vi "GEA2 HEWH Standard ERDs.vi"(8 "Error In":errorcluster, 10 "ERD Data Input":T1[](array[typedef]) {"ERD Number" format="%.0x"}, 11 "ERD Data  in":T2 {"ERD Therm Data"."EEV Possition" format="%0.0f"; "ERD Therm Data"."T6" format="%.1f"; "ERD Therm Data"."T2" format="%.1f"; "ERD Therm Data"."T3a" format="%.1f"; "ERD Therm Data"."T3b" format="%.1f"; "ERD Therm Data"."T4" format="%.1f"; "ERD Therm Data"."T5" format="%.1f"; "ERD Therm Data"."Current" format="%.1f"}) -> (0 "Error Out":errorcluster, 2 "ERD Data Output":T1[](array[typedef]) {"ERD Number" format="%.0x"}, 3 "ERD Data  out":T2 {"ERD Therm Data"."EEV Possition" format="%0.0f"; "ERD Therm Data"."T6" format="%.1f"; "ERD Therm Data"."T2" format="%.1f"; "ERD Therm Data"."T3a" format="%.1f"; "ERD Therm Data"."T3b" format="%.1f"; "ERD Therm Data"."T4" format="%.1f"; "ERD Therm Data"."T5" format="%.1f"; "ERD Therm Data"."Current" format="%.1f"})   [LabVIEW 2016]
uses:
  type defs/ERD Read Data Out.ctl
  type defs/HEWH ERD Data.ctl
  type defs/HEWH Faults.ctl
  type defs/HEWH Mixing Valve.ctl
  library/GEA2_Toolkit.lvlib
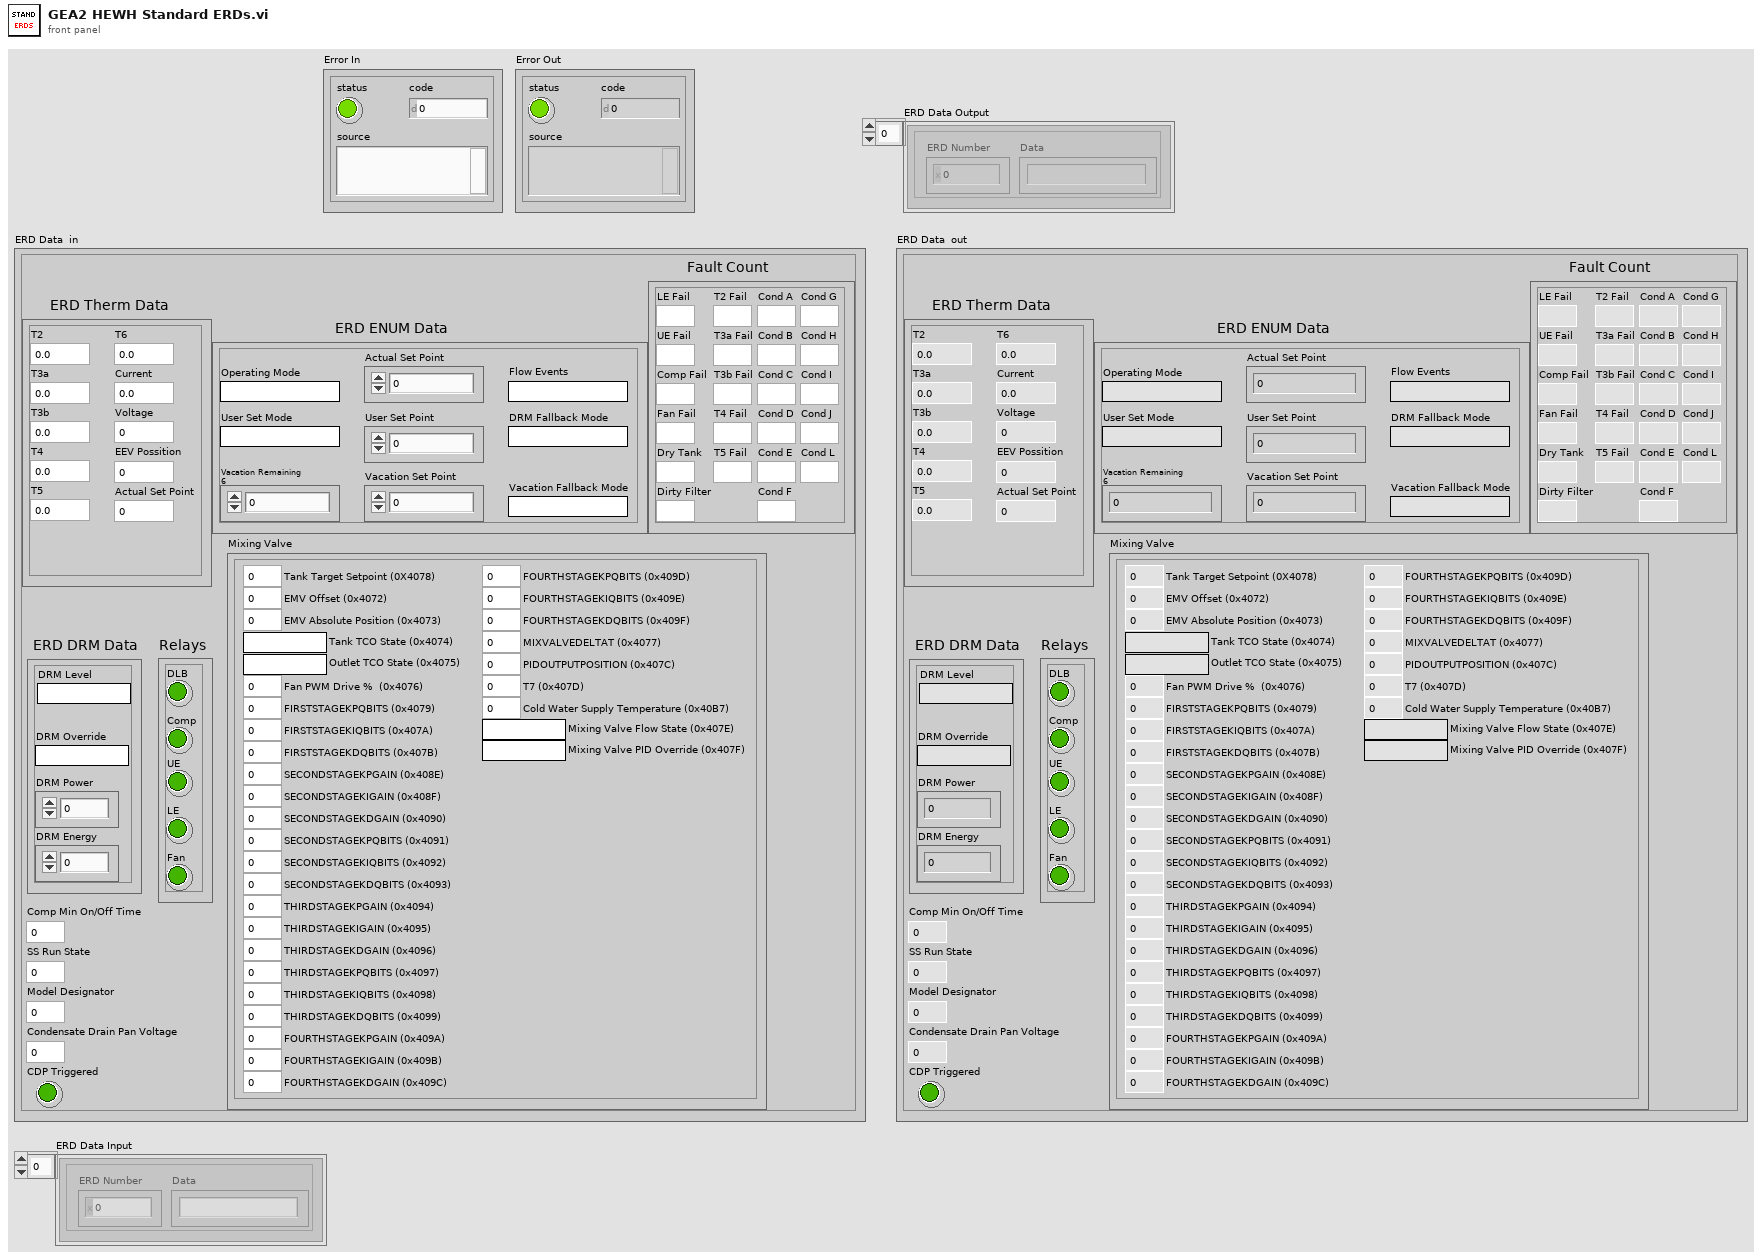
[diagram p1: front panel]
types:
  T1 = typedef "GEA2_Toolkit.lvlib/ERD Read Data Out.ctl" = cluster{"ERD Number":u16, "Data":string}
  T2 = typedef "HEWH ERD Data.ctl" = cluster{"ERD Therm Data":cluster{"T2":dbl, "T3a":dbl, "T3b":dbl, "T4":dbl, "T5":dbl, "T6":dbl, "Current":dbl, "Voltage":dbl, "EEV Possition":dbl, "Actual Set Point":dbl}, "ERD ENUM Data":cluster{"Actual Set Point":dbl, "Flow Events":string, "User Set Mode":string, "Operating Mode":string, "DRM Fallback Mode":string, "Vacation Fallback Mode":string, "User Set Point":dbl, "Vacation Set Point":dbl, "Vacation Remaining\n6":dbl}, "ERD DRM Data":cluster{"DRM Level":string, "DRM Override":string, "DRM Power":dbl, "DRM Energy":dbl}, "Fault Count":T3, "Relays":cluster{"DLB":bool, "Comp":bool, "UE":bool, "LE":bool, "Fan":bool}, "Comp Min On/Off Time":u16, "SS Run State":u16, "Condensate Drain Pan Voltage":u16, "CDP Triggered":bool, "Model Designator":u8, "Mixing Valve":T4}
  T3 = typedef "HEWH Faults.ctl" = cluster{"LE Fail":u32, "UE Fail":u32, "Comp Fail":u32, "T2 Fail":u32, "T3a Fail":u32, "T3b Fail":u32, "T4 Fail":u32, "T5 Fail":u32, "Cond A":u32, "Cond B":u32, "Cond C":u32, "Cond D":u32, "Cond E":u32, "Cond F":u32, "Cond G":u32, "Cond H":u32, "Cond I":u32, "Cond J":u32, "Cond L":u32, "Fan Fail":u32, "Dirty Filter":u32, "Dry Tank":u32}
  T4 = typedef "HEWH Mixing Valve.ctl" = cluster{"Tank Target Setpoint (0X4078)":dbl, "EMV Offset (0x4072)":dbl, "EMV Absolute Position (0x4073)":dbl, "Tank TCO State (0x4074)":string, "Outlet TCO State (0x4075)":string, "Fan PWM Drive %  (0x4076)":dbl, "FIRSTSTAGEKPQBITS (0x4079)":dbl, "FIRSTSTAGEKIQBITS (0x407A)":dbl, "FIRSTSTAGEKDQBITS (0x407B)":dbl, "SECONDSTAGEKPGAIN (0x408E)":dbl, "SECONDSTAGEKIGAIN (0x408F)":dbl, "SECONDSTAGEKDGAIN (0x4090)":dbl, "SECONDSTAGEKPQBITS (0x4091)":dbl, "SECONDSTAGEKIQBITS (0x4092)":dbl, "SECONDSTAGEKDQBITS (0x4093)":dbl, "THIRDSTAGEKPGAIN (0x4094)":dbl, "THIRDSTAGEKIGAIN (0x4095)":dbl, "THIRDSTAGEKDGAIN (0x4096)":dbl, "THIRDSTAGEKPQBITS (0x4097)":dbl, "THIRDSTAGEKIQBITS (0x4098)":dbl, "THIRDSTAGEKDQBITS (0x4099)":dbl, "FOURTHSTAGEKPGAIN (0x409A)":dbl, "FOURTHSTAGEKIGAIN (0x409B)":dbl, "FOURTHSTAGEKDGAIN (0x409C)":dbl, "FOURTHSTAGEKPQBITS (0x409D)":dbl, "FOURTHSTAGEKIQBITS (0x409E)":dbl, "FOURTHSTAGEKDQBITS (0x409F)":dbl, "MIXVALVEDELTAT (0x4077)":dbl, "PIDOUTPUTPOSITION (0x407C)":dbl, "T7 (0x407D)":dbl, "Cold Water Supply Temperature (0x40B7)":dbl, "Mixing Valve Flow State (0x407E)":string, "Mixing Valve PID Override (0x407F)":string}
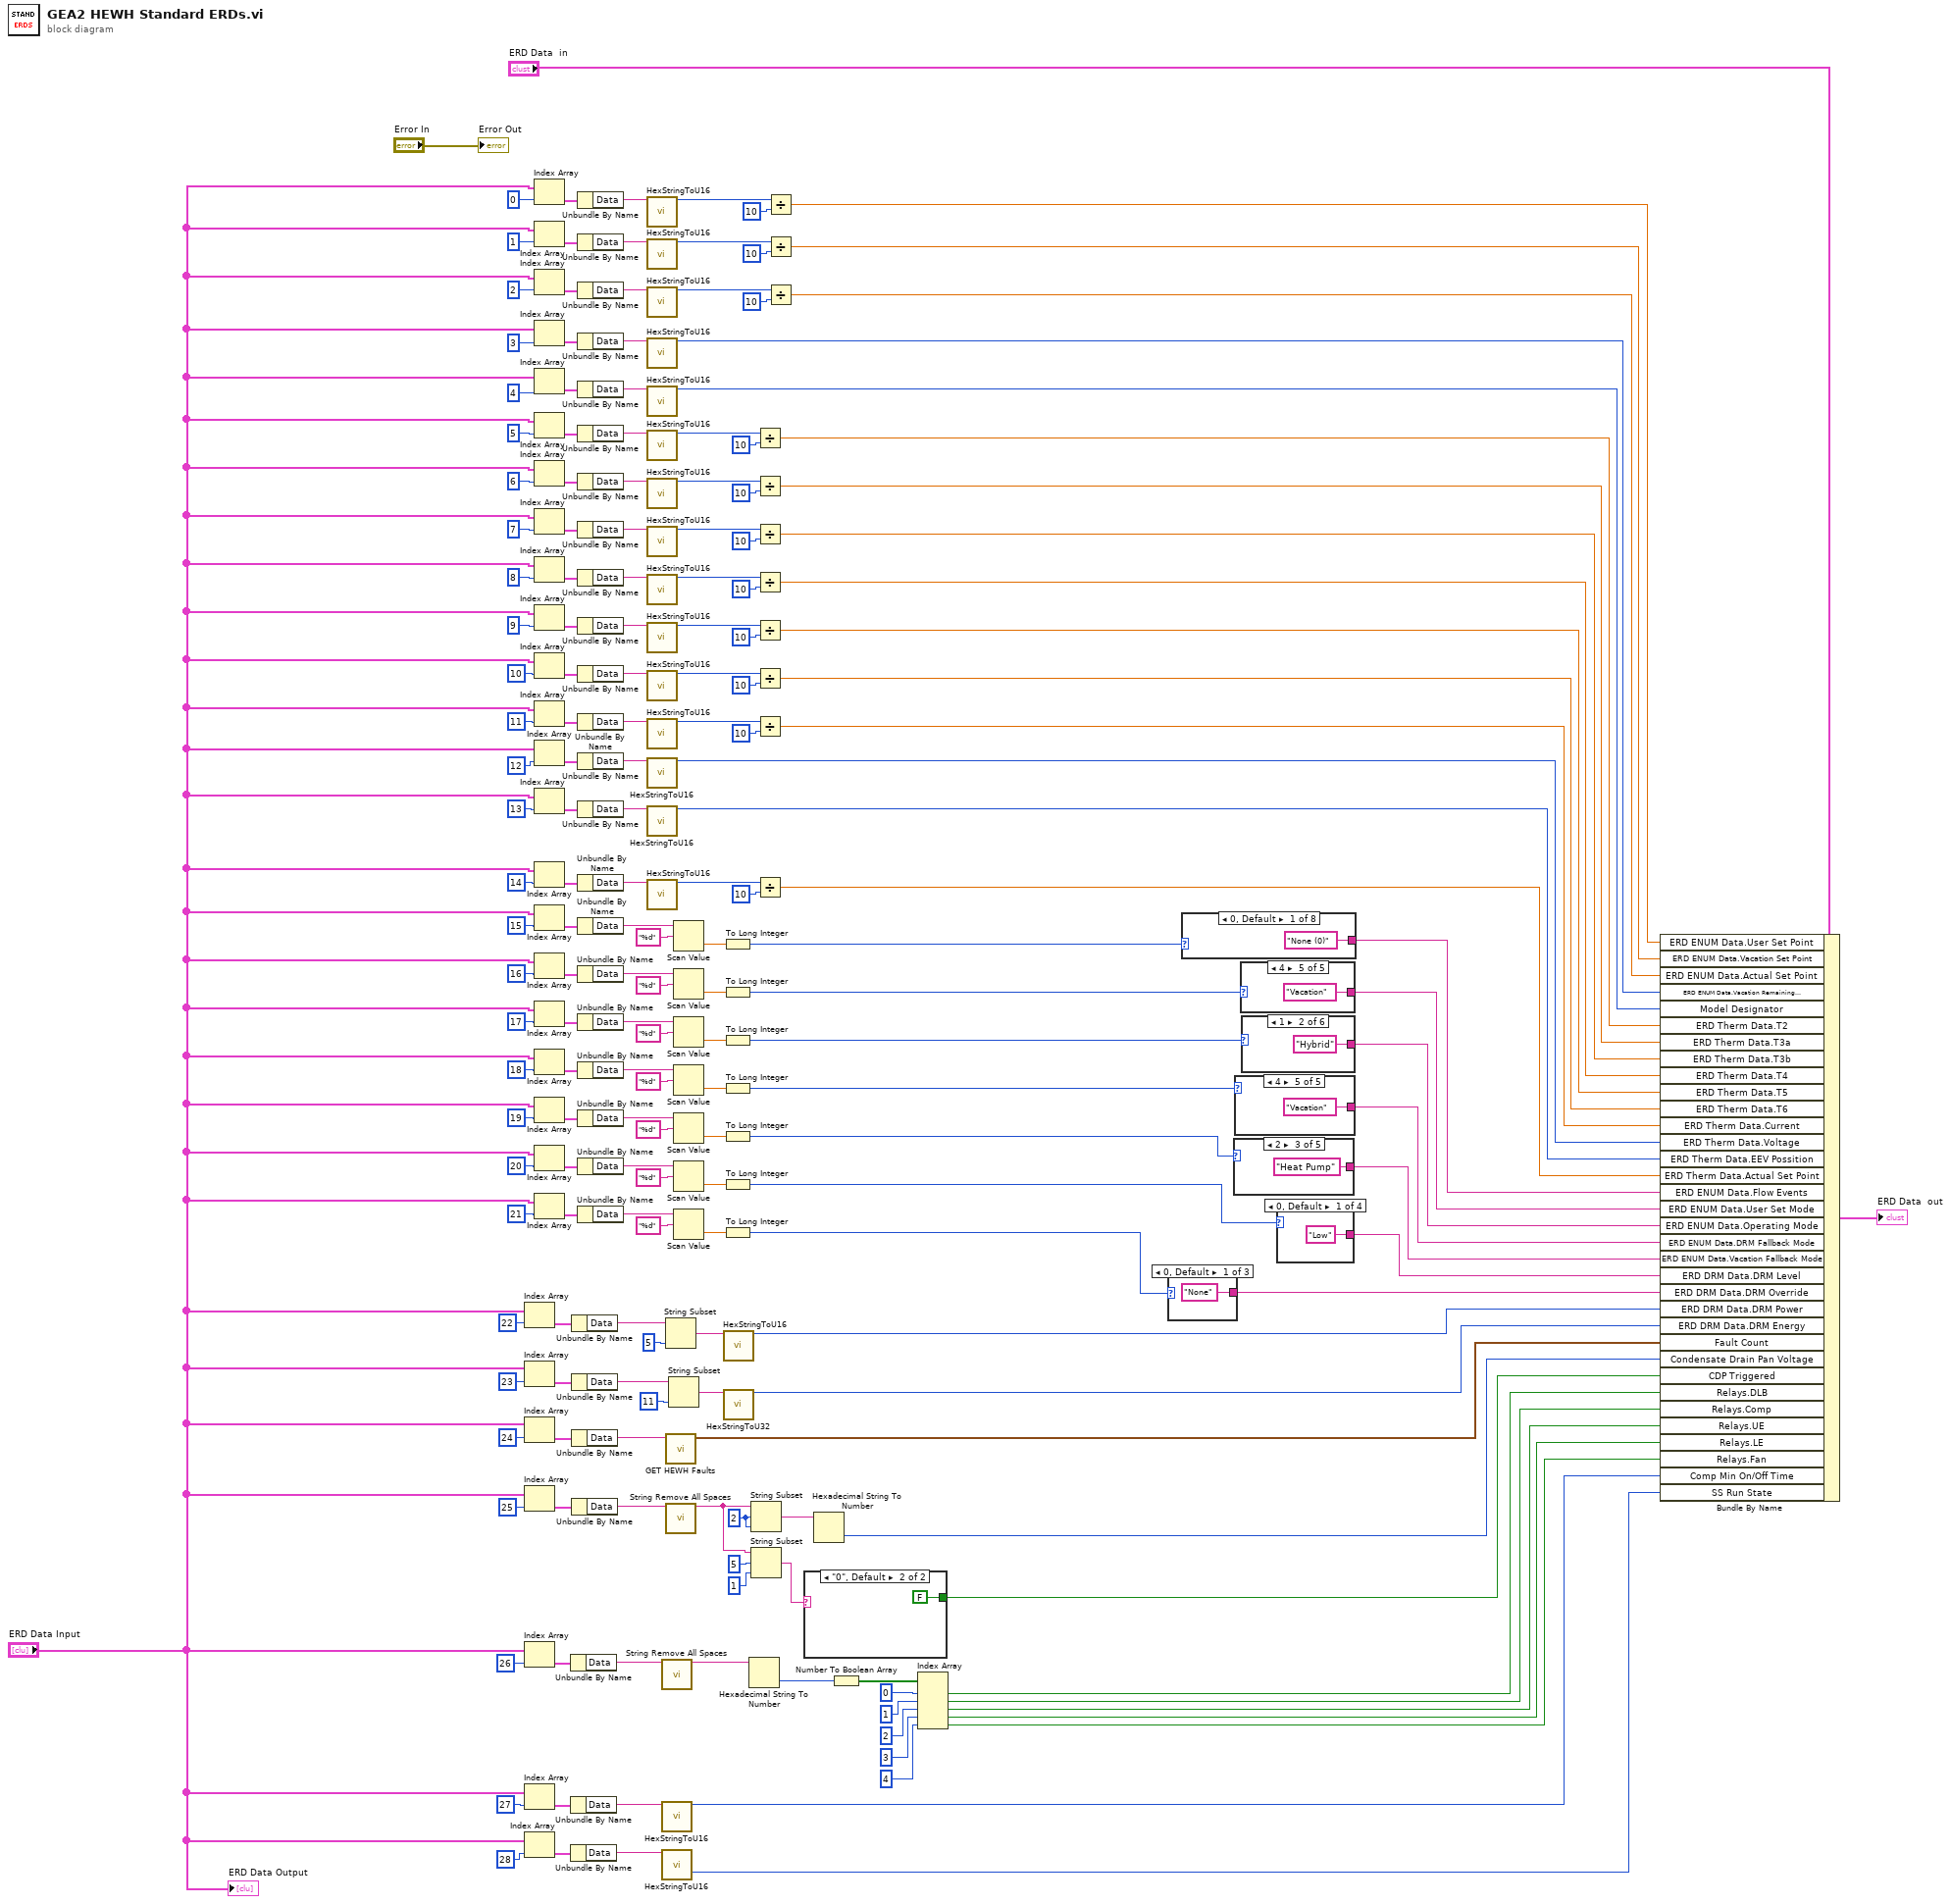
[diagram p0: block diagram]
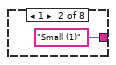
[diagram p2: hidden frame]
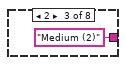
[diagram p3: hidden frame]
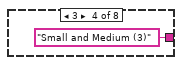
[diagram p4: hidden frame]
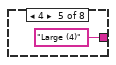
[diagram p5: hidden frame]
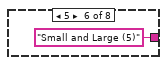
[diagram p6: hidden frame]
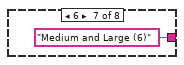
[diagram p7: hidden frame]
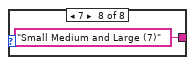
[diagram p8: hidden frame]
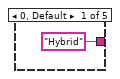
[diagram p9: hidden frame]
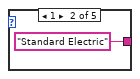
[diagram p10: hidden frame]
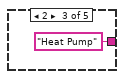
[diagram p11: hidden frame]
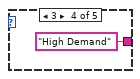
[diagram p12: hidden frame]
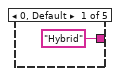
[diagram p13: hidden frame]
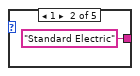
[diagram p14: hidden frame]
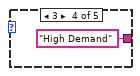
[diagram p15: hidden frame]
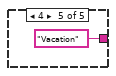
[diagram p16: hidden frame]
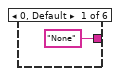
[diagram p17: hidden frame]
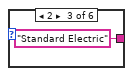
[diagram p18: hidden frame]
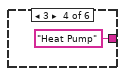
[diagram p19: hidden frame]
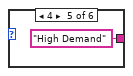
[diagram p20: hidden frame]
diagram:
  w134 = 2 ("length (rest)")
  n1 = Index Array(array="ERD Data Input", index=22) -> (element=w123:T1)
  n2 = Index Array(array="ERD Data Input", index=23) -> (element=w128:T1)
  n3 = Index Array(array="ERD Data Input", index=24) -> (element=w131:T1)
  n4 = Index Array(array="ERD Data Input", index=25) -> (element=w140:T1)
  n5 = Index Array(array="ERD Data Input", index=26) -> (element=w146:T1)
  n6 = Index Array(array="ERD Data Input", index=27) -> (element=w148:T1)
  n7 = Index Array(array="ERD Data Input", index=28) -> (element=w151:T1)
  n8 = Index Array(array="ERD Data Input", index=0) -> (element=w33:T1)
  n9 = Index Array(array="ERD Data Input", index=1) -> (element=w40:T1)
  n10 = Index Array(array="ERD Data Input", index=2) -> (element=w46:T1)
  n11 = Index Array(array="ERD Data Input", index=3) -> (element=w48:T1)
  n12 = Index Array(array="ERD Data Input", index=4) -> (element=w52:T1)
  n13 = Index Array(array="ERD Data Input", index=5) -> (element=w57:T1)
  n14 = Index Array(array="ERD Data Input", index=6) -> (element=w62:T1)
  n15 = Index Array(array="ERD Data Input", index=7) -> (element=w67:T1)
  n16 = Index Array(array="ERD Data Input", index=8) -> (element=w72:T1)
  n17 = Index Array(array="ERD Data Input", index=9) -> (element=w77:T1)
  n18 = Index Array(array="ERD Data Input", index=10) -> (element=w82:T1)
  n19 = Index Array(array="ERD Data Input", index=11) -> (element=w87:T1)
  n20 = Index Array(array="ERD Data Input", index=12) -> (element=w89:T1)
  n21 = Index Array(array="ERD Data Input", index=13) -> (element=w93:T1)
  n22 = Index Array(array="ERD Data Input", index=14) -> (element=w98:T1)
  n23 = Index Array(array="ERD Data Input", index=15) -> (element=w101:T1)
  n24 = Index Array(array="ERD Data Input", index=16) -> (element=w105:T1)
  n25 = Index Array(array="ERD Data Input", index=17) -> (element=w108:T1)
  n26 = Index Array(array="ERD Data Input", index=18) -> (element=w111:T1)
  n27 = Index Array(array="ERD Data Input", index=19) -> (element=w114:T1)
  n28 = Index Array(array="ERD Data Input", index=20) -> (element=w117:T1)
  n29 = Index Array(array="ERD Data Input", index=21) -> (element=w120:T1)
  n30 = Unbundle By Name(w146) -> ("Data"=w147:string)
  n31 = Unbundle By Name(w148) -> ("Data"=w149:string)
  n32 = Unbundle By Name(w151) -> ("Data"=w152:string)
  n33 = Unbundle By Name(w123) -> ("Data"=w124:string)
  n34 = Unbundle By Name(w128) -> ("Data"=w129:string)
  n35 = Unbundle By Name(w131) -> ("Data"=w132:string)
  n36 = Unbundle By Name(w140) -> ("Data"=w141:string)
  n37 = Unbundle By Name(w33) -> ("Data"=w34:string)
  n38 = Unbundle By Name(w40) -> ("Data"=w41:string)
  n39 = Unbundle By Name(w46) -> ("Data"=w43:string)
  n40 = Unbundle By Name(w48) -> ("Data"=w49:string)
  n41 = Unbundle By Name(w52) -> ("Data"=w51:string)
  n42 = Unbundle By Name(w57) -> ("Data"=w54:string)
  n43 = Unbundle By Name(w62) -> ("Data"=w61:string)
  n44 = Unbundle By Name(w67) -> ("Data"=w66:string)
  n45 = Unbundle By Name(w72) -> ("Data"=w69:string)
  n46 = Unbundle By Name(w77) -> ("Data"=w76:string)
  n47 = Unbundle By Name(w82) -> ("Data"=w79:string)
  n48 = Unbundle By Name(w87) -> ("Data"=w86:string)
  n49 = Unbundle By Name(w89) -> ("Data"=w90:string)
  n50 = Unbundle By Name(w93) -> ("Data"=w92:string)
  n51 = Unbundle By Name(w98) -> ("Data"=w95:string)
  n52 = Unbundle By Name(w101) -> ("Data"=w102:string)
  n53 = Unbundle By Name(w105) -> ("Data"=w103:string)
  n54 = Unbundle By Name(w108) -> ("Data"=w107:string)
  n55 = Unbundle By Name(w111) -> ("Data"=w109:string)
  n56 = Unbundle By Name(w114) -> ("Data"=w113:string)
  n57 = Unbundle By Name(w117) -> ("Data"=w115:string)
  n58 = Unbundle By Name(w120) -> ("Data"=w119:string)
  n59 = call "HexStringToU16.vi"("Input String"=w34) -> ("Number Out"=w31:u16)  [unwired: 14 in]
  n60 = call "HexStringToU16.vi"("Input String"=w41) -> ("Number Out"=w39:u16)  [unwired: 14 in]
  n61 = call "HexStringToU16.vi"("Input String"=w43) -> ("Number Out"=w45:u16)  [unwired: 14 in]
  n62 = call "HexStringToU16.vi"("Input String"=w49) -> ("Number Out"=w50:u16)  [unwired: 14 in]
  n63 = call "HexStringToU16.vi"("Input String"=w51) -> ("Number Out"=w53:u16)  [unwired: 14 in]
  n64 = call "HexStringToU16.vi"("Input String"=w54) -> ("Number Out"=w56:u16)  [unwired: 14 in]
  n65 = call "HexStringToU16.vi"("Input String"=w61) -> ("Number Out"=w59:u16)  [unwired: 14 in]
  n66 = call "HexStringToU16.vi"("Input String"=w66) -> ("Number Out"=w65:u16)  [unwired: 14 in]
  n67 = call "HexStringToU16.vi"("Input String"=w69) -> ("Number Out"=w70:u16)  [unwired: 14 in]
  n68 = call "HexStringToU16.vi"("Input String"=w76) -> ("Number Out"=w75:u16)  [unwired: 14 in]
  n69 = call "HexStringToU16.vi"("Input String"=w79) -> ("Number Out"=w80:u16)  [unwired: 14 in]
  n70 = call "HexStringToU16.vi"("Input String"=w86) -> ("Number Out"=w85:u16)  [unwired: 14 in]
  n71 = call "HexStringToU16.vi"("Input String"=w90) -> ("Number Out"=w91:u16)  [unwired: 14 in]
  n72 = call "HexStringToU16.vi"("Input String"=w92) -> ("Number Out"=w94:u16)  [unwired: 14 in]
  n73 = call "HexStringToU16.vi"("Input String"=w95) -> ("Number Out"=w96:u16)  [unwired: 14 in]
  n74 = call "String Remove All Spaces.vi"("Input String"=w147) -> ("Spaces Removed"=w145:string)  [unwired: 13 in, 1 out]
  n75 = call "HexStringToU16.vi"("Input String"=w149) -> ("Number Out"=w150:u16)  [unwired: 14 in]
  n76 = call "HexStringToU16.vi"("Input String"=w152) -> ("Number Out"=w153:u16)  [unwired: 14 in]
  n77 = String Subset(string=w124, length (rest)=5 ("length (rest)")) -> (substring=w121:string)  [unwired: 1 in]
  n78 = call "GET HEWH Faults.vi"("Data"=w132) -> ("Faults"=w133:T3)  [unwired: 10 in]
  n79 = call "String Remove All Spaces.vi"("Input String"=w141) -> ("Spaces Removed"=w137:string)  [unwired: 13 in, 1 out]
  n80 = String Subset(string=w129, length (rest)=11 ("length (rest)")) -> (substring=w126:string)  [unwired: 1 in]
  n81 = Scan Value(string=w102, format string="%d") -> (value=w184:dbl)  [unwired: 1 in, 1 out]
  n82 = Scan Value(string=w103, format string="%d") -> (value=w165:dbl)  [unwired: 1 in, 1 out]
  n83 = Scan Value(string=w107, format string="%d") -> (value=w175:dbl)  [unwired: 1 in, 1 out]
  n84 = Scan Value(string=w109, format string="%d") -> (value=w179:dbl)  [unwired: 1 in, 1 out]
  n85 = Scan Value(string=w113, format string="%d") -> (value=w181:dbl)  [unwired: 1 in, 1 out]
  n86 = Scan Value(string=w115, format string="%d") -> (value=w167:dbl)  [unwired: 1 in, 1 out]
  n87 = Scan Value(string=w119, format string="%d") -> (value=w171:dbl)  [unwired: 1 in, 1 out]
  n88 = To Long Integer(number=w184) -> (32bit integer=w183:i32)
  n89 = To Long Integer(number=w165) -> (32bit integer=w166:i32)
  n90 = To Long Integer(number=w175) -> (32bit integer=w174:i32)
  n91 = To Long Integer(number=w179) -> (32bit integer=w178:i32)
  n92 = To Long Integer(number=w181) -> (32bit integer=w177:i32)
  n93 = To Long Integer(number=w167) -> (32bit integer=w168:i32)
  n94 = To Long Integer(number=w171) -> (32bit integer=w172:i32)
  n95 = call "HexStringToU16.vi"("Input String"=w121) -> ("Number Out"=w125:u16)  [unwired: 14 in]
  n96 = call "HexStringToU32.vi"("Input String"=w126) -> ("Number Out"=w130:u32)  [unwired: 14 in]
  n97 = Hexadecimal String To Number(string=w145) -> (number=w144:u32)  [unwired: 2 in, 1 out]
  n98 = String Subset(string=w137, offset (0)=w134, length (rest)=w134) -> (substring=w139:string)
  n99 = String Subset(string=w137, offset (0)=5, length (rest)=1 ("length (rest)")) -> (substring=w136:string)
  n100 = Divide(x=w56, y=u16 10) -> (x/y=w58:dbl)
  n101 = Divide(x=w59, y=u16 10) -> (x/y=w63:dbl)
  n102 = Divide(x=w65, y=u16 10) -> (x/y=w68:dbl)
  n103 = Divide(x=w70, y=u16 10) -> (x/y=w73:dbl)
  n104 = Divide(x=w75, y=u16 10) -> (x/y=w78:dbl)
  n105 = Divide(x=w80, y=u16 10) -> (x/y=w83:dbl)
  n106 = Divide(x=w85, y=u16 10) -> (x/y=w88:dbl)
  n107 = Divide(x=w96, y=u16 10) -> (x/y=w99:dbl)
  n108 = Divide(x=w31, y=u16 10) -> (x/y=w37:dbl)
  n109 = Divide(x=w39, y=u16 10) -> (x/y=w42:dbl)
  n110 = Divide(x=w45, y=u16 10) -> (x/y=w47:dbl)
  n111 = case shown="\"0\", Default" w136 {
    tunnel: [TRUE FALSE] -> w143
    frame "1" {
    }
    frame "0", Default {
    }
  }
  n112 = Hexadecimal String To Number(string=w139) -> (number=w142:u32)  [unwired: 2 in, 1 out]
  n113 = Number To Boolean Array(number=w144) -> (Boolean array=w154:bool[])
  n114 = Index Array(array=w154, index #1=0 ("index"), index #2=1 ("index"), index #3=2 ("index"), index #4=3 ("index"), index #5=4 ("index")) -> (element #1=w160:bool, element #2=w161:bool, element #3=w162:bool, element #4=w163:bool, element #5=w164:bool)
  n115 = case shown="0, Default" w172 {
    tunnel: ["None" "Partial" "Full"] -> w173
    frame 0, Default {
    }
    frame 1 {
    }
    frame 2 {
    }
  }
  n116 = case shown="0, Default" w183 {
    tunnel: ["None (0)" "Small (1)" "Medium (2)" "Small and Medium (3)" "Large (4)" "Small and Large (5)" "Medium and Large (6)" "Small Medium and Large (7)"] -> w185
    frame 0, Default {
    }
    frame 1 {
    }
    frame 2 {
    }
    frame 3 {
    }
    frame 4 {
    }
    frame 5 {
    }
    frame 6 {
    }
    frame 7 {
    }
  }
  n117 = case shown="2" w177 {
    tunnel: ["Hybrid" "Standard Electric" "Heat Pump" "High Demand" "Vacation"] -> w182
    frame 0, Default {
    }
    frame 1 {
    }
    frame 2 {
    }
    frame 3 {
    }
    frame 4 {
    }
  }
  n118 = case shown="4" w178 {
    tunnel: ["Hybrid" "Standard Electric" "Heat Pump" "High Demand" "Vacation"] -> w180
    frame 0, Default {
    }
    frame 1 {
    }
    frame 2 {
    }
    frame 3 {
    }
    frame 4 {
    }
  }
  n119 = case shown="4" w166 {
    tunnel: ["Hybrid" "Standard Electric" "Heat Pump" "High Demand" "Vacation"] -> w170
    frame 0, Default {
    }
    frame 1 {
    }
    frame 2 {
    }
    frame 3 {
    }
    frame 4 {
    }
  }
  n120 = case shown="1" w174 {
    tunnel: ["None" "Hybrid" "Standard Electric" "Heat Pump" "High Demand" "Vacation"] -> w176
    frame 0, Default {
    }
    frame 1 {
    }
    frame 2 {
    }
    frame 3 {
    }
    frame 4 {
    }
    frame 5 {
    }
  }
  n121 = case shown="0, Default" w168 {
    tunnel: ["Low" "Medium" "High" "Critical"] -> w169
    frame 0, Default {
    }
    frame 1 {
    }
    frame 2 {
    }
    frame 3 {
    }
  }
  n122 = Bundle By Name(cluster="ERD Data  in", "ERD ENUM Data.User Set Point"=w37, "ERD ENUM Data.Vacation Set Point"=w42, "ERD ENUM Data.Actual Set Point"=w47, "ERD ENUM Data.Vacation Remaining\n6"=w50, "Model Designator"=w53, "ERD Therm Data.T2"=w58, "ERD Therm Data.T3a"=w63, "ERD Therm Data.T3b"=w68, "ERD Therm Data.T4"=w73, "ERD Therm Data.T5"=w78, "ERD Therm Data.T6"=w83, "ERD Therm Data.Current"=w88, "ERD Therm Data.Voltage"=w91, "ERD Therm Data.EEV Possition"=w94, "ERD Therm Data.Actual Set Point"=w99, "ERD ENUM Data.Flow Events"=w185, "ERD ENUM Data.User Set Mode"=w170, "ERD ENUM Data.Operating Mode"=w176, "ERD ENUM Data.DRM Fallback Mode"=w180, "ERD ENUM Data.Vacation Fallback Mode"=w182, "ERD DRM Data.DRM Level"=w169, "ERD DRM Data.DRM Override"=w173, "ERD DRM Data.DRM Power"=w125, "ERD DRM Data.DRM Energy"=w130, "Fault Count"=w133, "Condensate Drain Pan Voltage"=w142, "CDP Triggered"=w143, "Relays.DLB"=w160, "Relays.Comp"=w161, "Relays.UE"=w162, "Relays.LE"=w163, "Relays.Fan"=w164, "Comp Min On/Off Time"=w150, "SS Run State"=w153) -> (→"ERD Data  out":T2)
  "Error Out" <- "Error In"
  "ERD Data Output" <- "ERD Data Input"
